vi "Autonomous Independent.vi"   [LabVIEW 2013]
doc: "This VI is called when autonomous begins, and will automatically be terminated when autonomous ends. You can carry out timed or sensor driven robot movement independently without needing to return to the caller."
uses:
  Robot Global Data.vi
panel:
  # "Be sure to right-click and choose Data Operations>>Make Current Value default if you want to save the array values with the VI"
types:
  T1 = cluster{"X":dbl, "Y":dbl, "Ending Angle":dbl, "Use Ending Angle?":bool}
  T2 = typedef "WPI_EncoderDevRef.ctl" = cluster{"DevStatus":errorcluster, "EncoderIndex":T3, "CounterIndex":T4, "DistancePerCount":dbl, "Decoding Type":T5}
  T3 = typedef "FPGA_EncoderIdx.ctl" = enum8{"Enc 0", "Enc 1", "Enc 2", "Enc 3", "Invalid"}
  T4 = typedef "FPGA_CounterCtrSystemIndex.ctl" = enum8{"Ctr 0", "Ctr 1", "Ctr 2", "Ctr 3", "Ctr 4", "Ctr 5", "Ctr 6", "Ctr 7", "Invalid"}
  T5 = typedef "WPI_EncoderType.ctl" = enum16{"1x", "2x", "4x"}
  T6 = typedef "WPI_MotorControlDeviceRef.ctl" = cluster{"DeviceStatus":errorcluster, "Type":enum16{"PWM", "CAN"}, "PWM":cluster{"Digital Module":T7, "PWM Channel":T8, "DeadBand":T9}, "CAN":cluster{"Device Number":u8, "Control Mode":T10, "Semaphore":T11, "Max Vout":dbl}, "Invert":bool, "TransformRef":T12, "InvTransformRef":T12}
  T7 = typedef "FPGA_TypedefDigitalModule.ctl" = enum16{"Digital Module 1", "Digital Module 2"}
  T8 = typedef "FPGA_DIOPWMChannel.ctl" = enum8{"PWM 1", "PWM 2", "PWM 3", "PWM 4", "PWM 5", "PWM 6", "PWM 7", "PWM 8", "PWM 9", "PWM 10", "Invalid"}
  T9 = typedef "WPI_PWMDeadband.ctl" = cluster{"Name":string, "maxPositivePwm":i32, "minPositivePwm":i32, "centerPwm":i32, "maxNegativePwm":i32, "minNegativePwm":i32, "angularRange":u16}
  T10 = typedef "WPI_CANJaguar_ControlMode.ctl" = enum8{"Percent VBus", "Current", "Speed", "Position", "Voltage"}
  T11 = typedef "Semaphore RefNum" = refnum<k1>
  T12 = typedef "WPI_PWMTransform_ConPane.ctl" = refnum<vi>
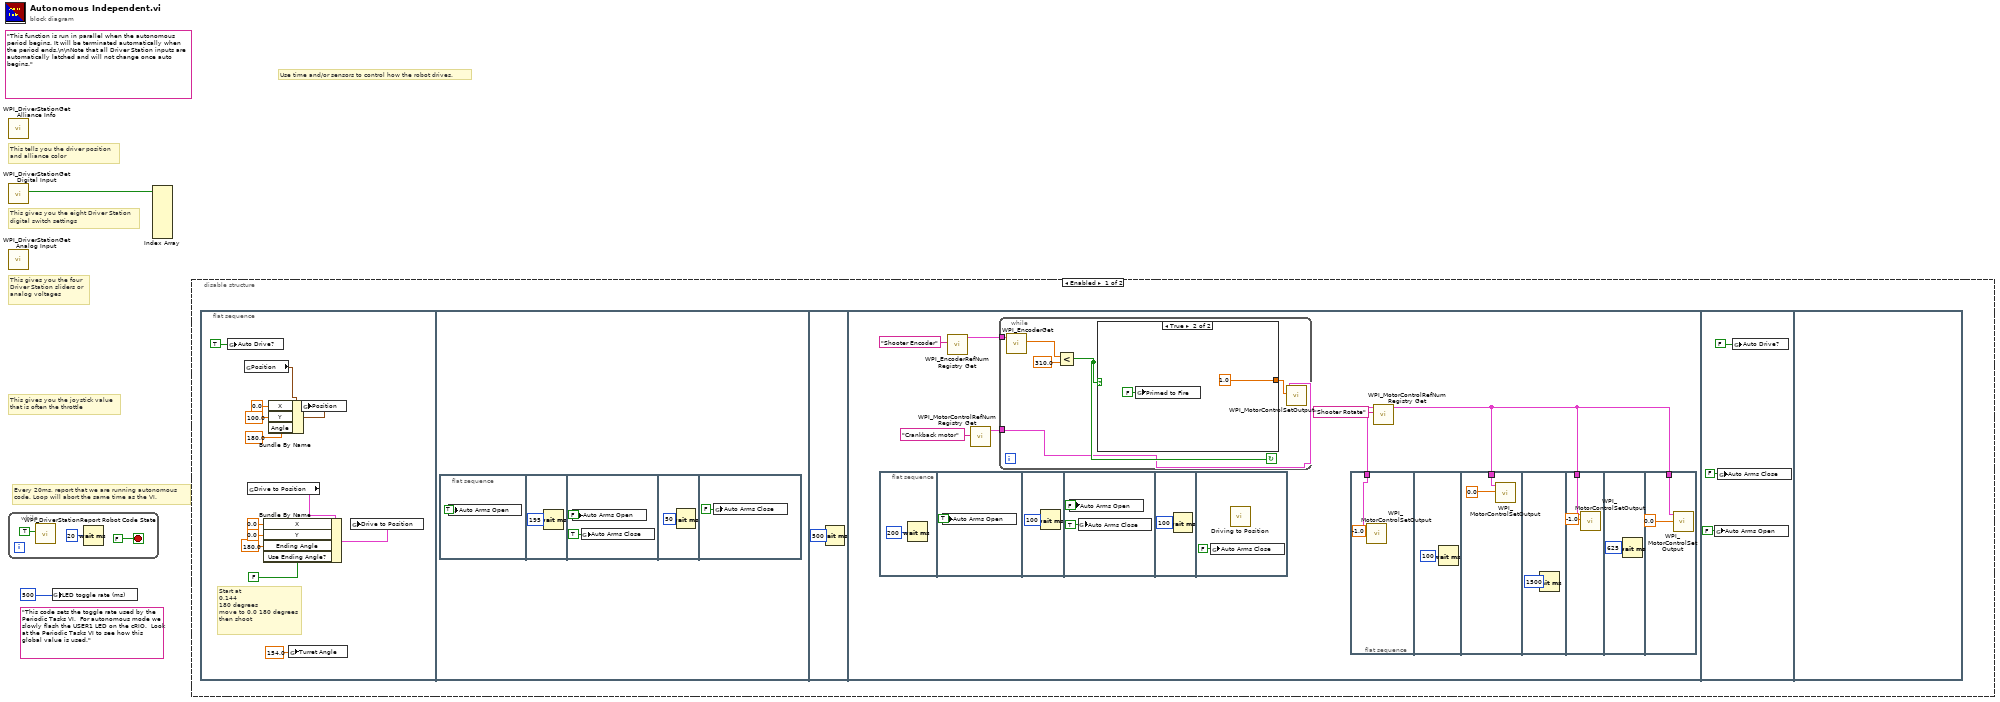
[diagram p0: block diagram]
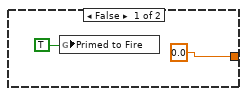
[diagram p2: hidden frame]
diagram:
  (unwired) "This code sets the toggle rate used by the Periodic Tasks VI.  For autonomous mode we slowly flash the USER1 LED on the cRIO.  Look at the Periodic Tasks VI to see how this global value is used."
  (unwired) "This function is run in parallel when the autonomous period begins. It will be terminated automatically when the period ends.\n\nNote that all Driver Station inputs are automatically latched and will not change once auto begins."
  # "Every 20ms, report that we are running autonomous\ncode. Loop will abort the same time as the VI."
  # "This gives you the joystick value\nthat is often the throttle"
  # "Use time and/or sensors to control how the robot drives."
  # "This tells you the driver position\nand alliance color"
  # "This gives you the eight Driver Station\ndigital switch settings"
  # "This gives you the four\nDriver Station sliders or\nanalog voltages"
  n1 = while {
    stop <- FALSE stop-if-true
    n2 = call <vilib>:"WPI_DriverStationReport Robot Code State.vi"("Autonomous"=TRUE) -> ()  [unwired: 10 in, 1 out]
    n3 = Wait (ms)(milliseconds to wait=u32 20) -> ()  [unwired: 1 out]
  }
  n4 = call <vilib>:"WPI_DriverStationGet Alliance Info.vi"() -> ()  [unwired: 12 out]
  n5 = call <vilib>:"WPI_DriverStationGet Digital Input.vi"() -> ("Driver Station Digital Input (1-8)"=w2:bool[])  [unwired: 11 out]
  n6 = call <vilib>:"WPI_DriverStationGet Analog Input.vi"() -> ()  [unwired: 12 out]
  n7 = global write "Robot Global Data.vi" "LED toggle rate (ms)"(u32 500 ("LED ms toggle rate")) -> ()
  n8 = Index Array(array=w2) -> ()  [unwired: 8 in, 8 out]
  n9 = disable-structure shown="Enabled" {
    frame Enabled {
      n10 = flat-sequence {
        frame #0 {
          # "Start at \n0,144\n180 degrees\nmove to 0,0 180 degrees\nthen shoot"
          n11 = global write "Robot Global Data.vi" "Auto Drive?"(TRUE) -> ()
          n12 = global read "Robot Global Data.vi" "Position"() -> (w16:cluster{"X":dbl, "Y":dbl, "Angle":dbl})
          n13 = global read "Robot Global Data.vi" "Drive to Position"() -> (w14:T1)
          n14 = Bundle By Name(cluster=w14, "X"=0.0, "Y"=0.0, "Ending Angle"=180.0, "Use Ending Angle?"=FALSE) -> (w15:T1)
          n15 = Bundle By Name(cluster=w16, "X"=0.0, "Y"=100.0, "Angle"=180.0) -> (w17:cluster{"X":dbl, "Y":dbl, "Angle":dbl})
          n16 = global write "Robot Global Data.vi" "Turret Angle"(154.0 ("Turret Angle")) -> ()
          n17 = global write "Robot Global Data.vi" "Position"(w17) -> ()
          n18 = global write "Robot Global Data.vi" "Drive to Position"(w15) -> ()
        }
        frame #1 {
          n19 = flat-sequence {
            frame #0 {
              n20 = global write "Robot Global Data.vi" "Auto Arms Open"(TRUE ("Auto Arms Open")) -> ()
            }
            frame #1 {
              n21 = Wait (ms)(milliseconds to wait=u32 195) -> ()  [unwired: 1 out]
            }
            frame #2 {
              n22 = global write "Robot Global Data.vi" "Auto Arms Open"(FALSE ("Auto Arms Open")) -> ()
              n23 = global write "Robot Global Data.vi" "Auto Arms Close"(TRUE ("Auto Arms Close")) -> ()
            }
            frame #3 {
              n24 = Wait (ms)(milliseconds to wait=u32 50) -> ()  [unwired: 1 out]
            }
            frame #4 {
              n25 = global write "Robot Global Data.vi" "Auto Arms Close"(FALSE ("Auto Arms Close")) -> ()
            }
          }
        }
        frame #2 {
          n26 = Wait (ms)(milliseconds to wait=u32 500) -> ()  [unwired: 1 out]
        }
        frame #3 {
          n27 = flat-sequence {
            frame #0 {
              n28 = Wait (ms)(milliseconds to wait=u32 200) -> ()  [unwired: 1 out]
            }
            frame #1 {
              n29 = global write "Robot Global Data.vi" "Auto Arms Open"(TRUE ("Auto Arms Open")) -> ()
            }
            frame #2 {
              n30 = Wait (ms)(milliseconds to wait=u32 100) -> ()  [unwired: 1 out]
            }
            frame #3 {
              n31 = global write "Robot Global Data.vi" "Auto Arms Open"(FALSE ("Auto Arms Open")) -> ()
              n32 = global write "Robot Global Data.vi" "Auto Arms Close"(TRUE ("Auto Arms Close")) -> ()
            }
            frame #4 {
              n33 = Wait (ms)(milliseconds to wait=u32 100) -> ()  [unwired: 1 out]
            }
            frame #5 {
              n34 = global write "Robot Global Data.vi" "Auto Arms Close"(FALSE ("Auto Arms Close")) -> ()
              n35 = call "Driving to Position.vi"() -> ()  [unwired: 12 in]
            }
          }
          n36 = call <vilib>:"WPI_EncoderRefNum Registry Get.vi"("refnum name"="Shooter Encoder") -> ("EncoderDevRef"=w28:T2)  [unwired: 9 in, 1 out]
          n37 = call <vilib>:"WPI_MotorControlRefNum Registry Get.vi"("refnum name"="Crankback motor") -> ("MotorControlDevRef"=w26:T6)  [unwired: 9 in, 1 out]
          n38 = while {
            tunnel: w28 -> [w34]
            tunnel: w26 -> [w32]
            stop <- w35 continue-if-true
            n39 = call <vilib>:"WPI_EncoderGet.vi"("EncoderDevRef"=w34) -> ("Distance"=w36:dbl)  [unwired: 5 in, 5 out]
            n40 = Less?(x=w36, y=310.0) -> (x < y?=w35:bool)
            n41 = case shown="True" w35 {
              tunnel: [0.0 1.0] -> w33
              frame False {
                n42 = global write "Robot Global Data.vi" "Primed to Fire"(TRUE ("Locked")) -> ()
              }
              frame True {
                n43 = global write "Robot Global Data.vi" "Primed to Fire"(FALSE ("Locked")) -> ()
              }
            }
            n44 = call <vilib>:"WPI_MotorControlSetOutput.vi"("Output"=w33, "MotorControlDevRef"=w32) -> ()  [unwired: 7 in, 3 out]
          }
          n45 = flat-sequence {
            tunnel: w30 -> [w49]
            tunnel: w30 -> [w53]
            tunnel: w30 -> [w55]
            tunnel: w30 -> [w58]
            frame #0 {
              n46 = call <vilib>:"WPI_MotorControlSetOutput.vi"("Output"=-1.0, "MotorControlDevRef"=w49) -> ()  [unwired: 7 in, 3 out]
            }
            frame #1 {
              n47 = Wait (ms)(milliseconds to wait=u32 100) -> ()  [unwired: 1 out]
            }
            frame #2 {
              n48 = call <vilib>:"WPI_MotorControlSetOutput.vi"("Output"=0.0, "MotorControlDevRef"=w53) -> ()  [unwired: 7 in, 3 out]
            }
            frame #3 {
              n49 = Wait (ms)(milliseconds to wait=u32 1500) -> ()  [unwired: 1 out]
            }
            frame #4 {
              n50 = call <vilib>:"WPI_MotorControlSetOutput.vi"("Output"=-1.0, "MotorControlDevRef"=w55) -> ()  [unwired: 7 in, 3 out]
            }
            frame #5 {
              n51 = Wait (ms)(milliseconds to wait=u32 625) -> ()  [unwired: 1 out]
            }
            frame #6 {
              n52 = call <vilib>:"WPI_MotorControlSetOutput.vi"("Output"=0.0, "MotorControlDevRef"=w58) -> ()  [unwired: 7 in, 3 out]
            }
          }
          n53 = call <vilib>:"WPI_MotorControlRefNum Registry Get.vi"("refnum name"="Shooter Rotate") -> ("MotorControlDevRef"=w30:T6)  [unwired: 9 in, 1 out]
        }
        frame #4 {
          n54 = global write "Robot Global Data.vi" "Auto Arms Open"(FALSE ("Auto Arms Close")) -> ()
          n55 = global write "Robot Global Data.vi" "Auto Arms Close"(FALSE ("Auto Arms Close")) -> ()
          n56 = global write "Robot Global Data.vi" "Auto Drive?"(FALSE) -> ()
        }
        frame #5 {
        }
      }
    }
    frame Disabled {
    }
  }
